vi "StepGlobal.vi"(10 "Action (Get)":enum16{"Clear", "Append", "Set", "Get"}(ring)=enum."Get", 11 "AutoScriptSteps in":T1(array[cluster])) -> (3 "AutoScriptSteps out":T1(array[cluster]))   [LabVIEW 2015]
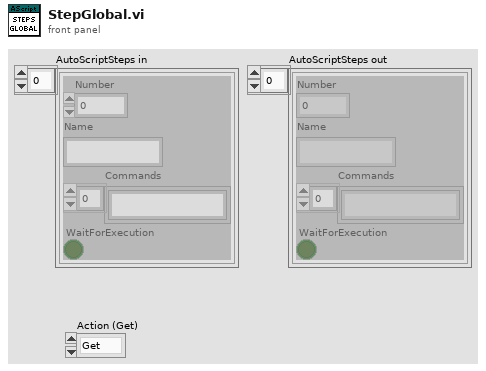
[diagram p1: front panel]
types:
  T1 = cluster{"Number":i32, "Name":string, "Commands":string[], "WaitForExecution":bool}[]
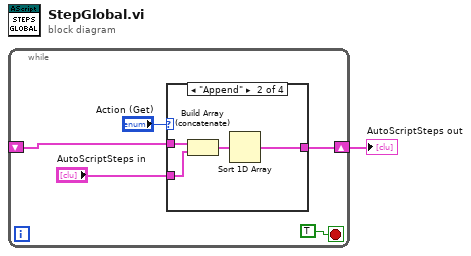
[diagram p0: block diagram]
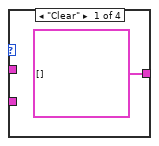
[diagram p2: hidden frame]
diagram:
  n1 = while {
    shift-right: [w3] -> w1
    shift-left: _ -> [w2]
    stop <- TRUE stop-if-true
    n2 = case shown="\"Append\"" "Action (Get)" {
      tunnel: "AutoScriptSteps in" -> [_ w10 w12 _]
      tunnel: [T1 [] ("AutoScriptSteps in") w8 w12 w13] -> w3
      tunnel: w2 -> [_ w11 _ w13]
      frame "Clear" {
      }
      frame "Append" {
        n3 = Build Array (concatenate)(w11, w10) -> (w9:T1)
        n4 = Sort 1D Array(array=w9) -> (sorted array=w8:T1)
      }
      frame "Set" {
      }
      frame "Get", Default {
      }
    }
  }
  "AutoScriptSteps out" <- w1
